vi "Pi-Drive - Drive Sine Smooth (SubVI).vi"(0 "High Gear":bool, 1 "High Gear Input Non-Linearity {-1...1}":dbl=1.0, 9 "Low Gear Input Non-Linearity {-1...1}":dbl=0.5, 11 "Increase Curve":dbl=2.5, 12 "Input":dbl) -> (3 "High Gear Non-Linearity Output":dbl=0.5, 4 "High Gear Output":bool, 10 "Low Gear Non-Linearity  Output":dbl=0.5, 15 "Smoothed Output":dbl)   [LabVIEW 2019]
panel:
  # "Inputs"
  # "Controls"
  # "Indicators"
  # "Outputs"
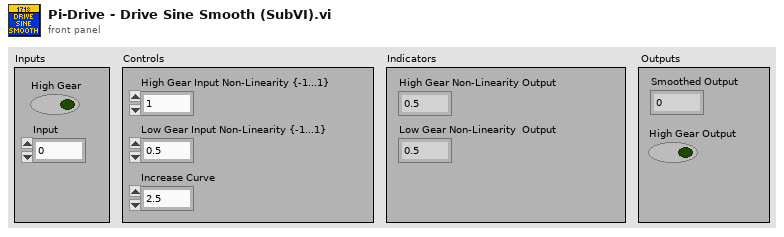
[diagram p1: front panel]
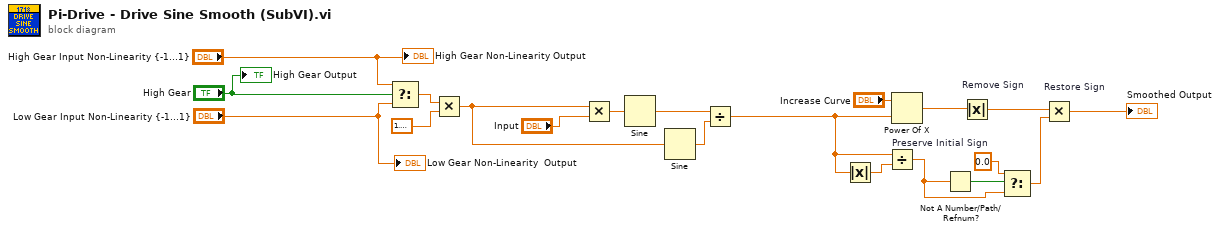
[diagram p0: block diagram]
diagram:
  n1 = Select(t="High Gear Input Non-Linearity {-1...1}", s="High Gear", f="Low Gear Input Non-Linearity {-1...1}") -> (s? t:f=w13:dbl)
  n2 = Multiply(x=w13, y=1.5707963267948966) -> (x*y=w20:dbl)
  n3 = Multiply(x=w20, y="Input") -> (x*y=w17:dbl)
  n4 = Sine(x=w17) -> (sin(x)=w18:dbl)
  n5 = Sine(x=w20) -> (sin(x)=w19:dbl)
  n6 = Divide(x=w18, y=w19) -> (x/y=w2:dbl)
  n7 = Absolute Value(x=w2) -> (abs(x)=w9:dbl)
  n8 = Divide "Preserve Initial Sign"(x=w2, y=w9) -> (x/y=w1:dbl)
  n9 = Power Of X(1:w2, 2:"Increase Curve") -> (0:w7:dbl)
  n10 = Not A Number/Path/Refnum?(number/path/refnum=w1) -> (NaN/Path/Refnum?=w5:bool)
  n11 = Absolute Value "Remove Sign"(x=w7) -> (abs(x)=w6:dbl)
  n12 = Select(t=0.0 ("f"), s=w5, f=w1) -> (s? t:f=w4:dbl)
  n13 = Multiply "Restore Sign"(x=w6, y=w4) -> (x*y=→"Smoothed Output":dbl)
  "High Gear Non-Linearity Output" <- "High Gear Input Non-Linearity {-1...1}"
  "Low Gear Non-Linearity  Output" <- "Low Gear Input Non-Linearity {-1...1}"
  "High Gear Output" <- "High Gear"
